vi "Rotate Image.vi"(10 "Degrees":dbl, 11 "Image":T1) -> (3 "Rotated Image":T1)   [LabVIEW 2020, in "User Interface.lvlib"]
uses:
  User Interface.lvlib
  <vilib>/picture/picture.llb/imagedata.ctl
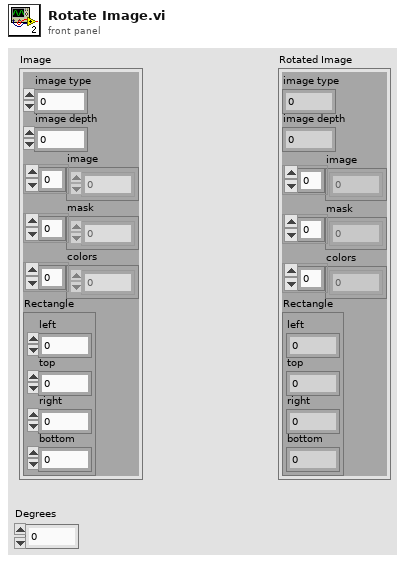
[diagram p1: front panel]
types:
  T1 = typedef "imagedata.ctl" = cluster{"image type":i32, "image depth":i32, "image":u8[], "mask":u8[], "colors":u32[], "Rectangle":cluster{"left":i16, "top":i16, "right":i16, "bottom":i16}}
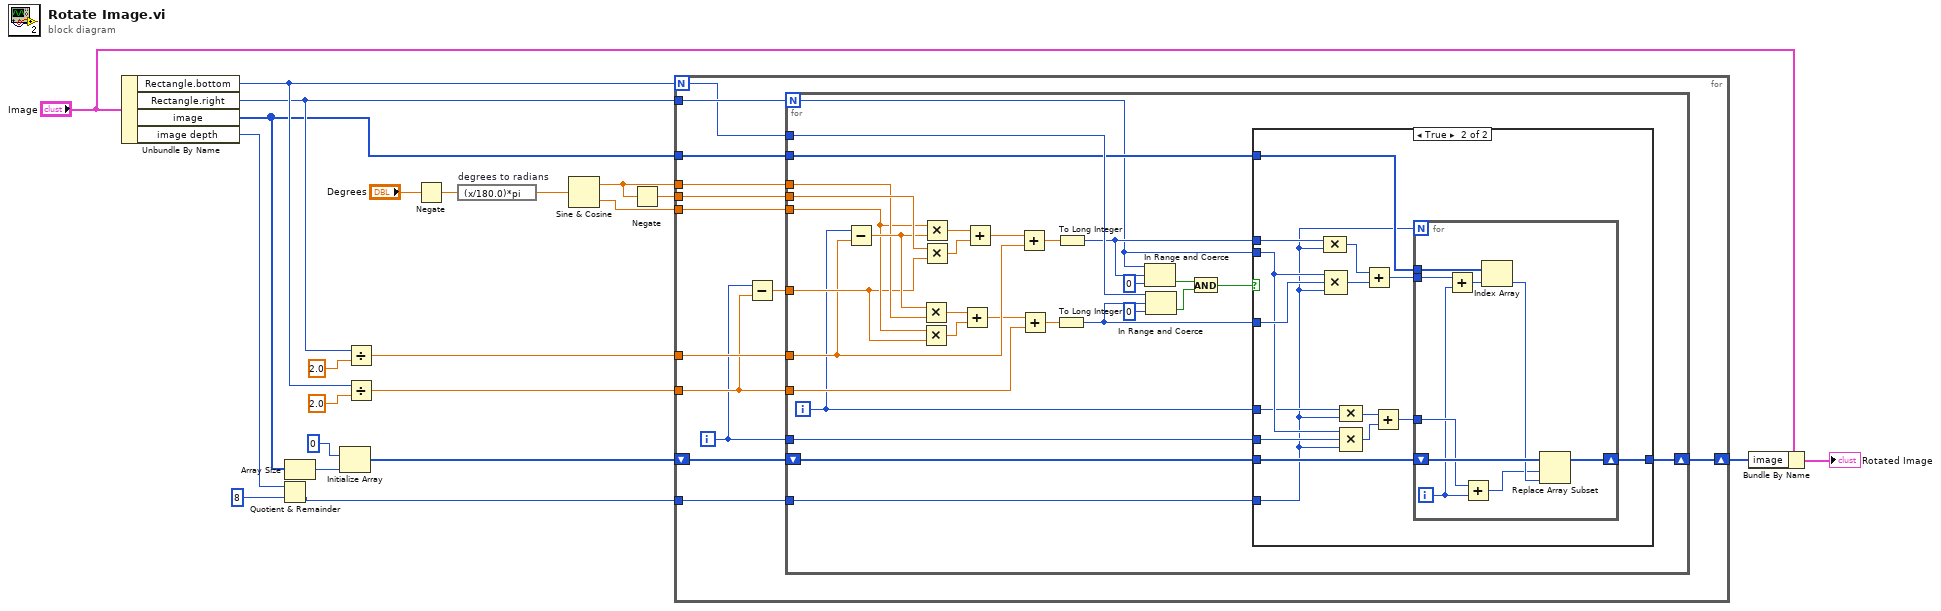
[diagram p0: block diagram]
diagram:
  n1 = Unbundle By Name("Image") -> ("Rectangle.bottom"=w22:i16, "Rectangle.right"=w21:i16, "image"=w18:u8[], "image depth"=w15:i32)
  n2 = Quotient & Remainder(x=w15, y=8) -> (floor(x/y)=w14:i32)  [unwired: 1 out]
  n3 = Array Size(array=w18) -> (size(s)=w20:i32)
  n4 = Initialize Array(u8 0, w20) -> (w17:u8[])
  n5 = Divide(x=w21, y=2.0) -> (x/y=w11:dbl)
  n6 = Divide(x=w22, y=2.0) -> (x/y=w10:dbl)
  n7 = Negate(x="Degrees") -> (-x=w5:dbl)
  n8 = expression code="(x/180.0)*pi" "degrees to radians"(w5) -> (w9:dbl)
  n9 = Sine & Cosine(0:w9) -> (1:w6:dbl, 2:w8:dbl)
  n10 = Negate(x=w6) -> (-x=w7:dbl)
  n11 = for {
    N: w22 -> [w27]
    tunnel: w21 -> [w35]
    tunnel: w18 -> [w34]
    tunnel: w11 -> [w33]
    tunnel: w10 -> [w32]
    tunnel: w8 -> [w30]
    tunnel: w7 -> [w29]
    tunnel: w6 -> [w28]
    shift-right: [w24] -> w4
    shift-left: w17 -> [w25]
    tunnel: w14 -> [w23]
    i -> [w26]
    n12 = Subtract(x=w26, y=w32) -> (x-y=w31:dbl)
    n13 = for {
      N: w35 -> [w44]
      tunnel: w34 -> [w47]
      tunnel: w33 -> [w55]
      tunnel: w32 -> [w53]
      tunnel: w31 -> [w59]
      tunnel: w30 -> [w60]
      tunnel: w29 -> [w65]
      tunnel: w28 -> [w61]
      tunnel: w27 -> [w50]
      tunnel: w26 -> [w42]
      shift-right: [w40] -> w24
      shift-left: w25 -> [w41]
      tunnel: w23 -> [w37]
      i -> [w43]
      n14 = Subtract(x=w43, y=w55) -> (x-y=w62:dbl)
      n15 = Multiply(x=w62, y=w61) -> (x*y=w58:dbl)
      n16 = Multiply(x=w60, y=w59) -> (x*y=w57:dbl)
      n17 = Multiply(x=w60, y=w62) -> (x*y=w64:dbl)
      n18 = Multiply(x=w65, y=w59) -> (x*y=w63:dbl)
      n19 = Add(x=w58, y=w57) -> (x+y=w54:dbl)
      n20 = Add(x=w64, y=w63) -> (x+y=w56:dbl)
      n21 = Add(x=w56, y=w55) -> (x+y=w52:dbl)
      n22 = Add(x=w54, y=w53) -> (x+y=w51:dbl)
      n23 = To Long Integer(number=w51) -> (32bit integer=w45:i32)
      n24 = To Long Integer(number=w52) -> (32bit integer=w46:i32)
      n25 = In Range and Coerce(upper limit=w44, x=w46, lower limit=0) -> (In Range?=w49:bool)  [unwired: 1 out]
      n26 = In Range and Coerce(upper limit=w50, x=w45, lower limit=0) -> (In Range?=w48:bool)  [unwired: 1 out]
      n27 = And(x=w49, y=w48) -> (x .and. y?=w36:bool)
      n28 = case shown="True" w36 {
        tunnel: w47 -> [_ w81]
        tunnel: w46 -> [_ w78]
        tunnel: w45 -> [_ w80]
        tunnel: w44 -> [_ w76]
        tunnel: w43 -> [_ w73]
        tunnel: w42 -> [_ w75]
        tunnel: w41 -> [w66 w72]
        tunnel: [w66 w71] -> w40
        tunnel: w37 -> [_ w67]
        frame False {
        }
        frame True {
          n29 = Compound Arithmetic op=MULTIPLY(w78, w67) -> (w68:i32)
          n30 = Compound Arithmetic op=MULTIPLY(w76, w80, w67) -> (w79:i32)
          n31 = Compound Arithmetic op=MULTIPLY(w73, w67) -> (w69:i32)
          n32 = Compound Arithmetic op=MULTIPLY(w76, w75, w67) -> (w74:i32)
          n33 = Add(x=w68, y=w79) -> (x+y=w77:i32)
          n34 = Add(x=w69, y=w74) -> (x+y=w70:i32)
          n35 = for {
            N: w67 -> [_]
            tunnel: w81 -> [w90]
            tunnel: w77 -> [w84]
            tunnel: w70 -> [w86]
            shift-right: [w88] -> w71
            shift-left: w72 -> [w89]
            i -> [w83]
            n36 = Add(x=w84, y=w83) -> (x+y=w82:i32)
            n37 = Add(x=w86, y=w83) -> (x+y=w85:i32)
            n38 = Index Array(array=w90, index=w82) -> (element=w87:u8)
            n39 = Replace Array Subset(array=w89, new element=w87, index=w85) -> (w88:u8[])
          }
        }
      }
    }
  }
  n40 = Bundle By Name(cluster="Image", "image"=w4) -> (→"Rotated Image":T1)
